vi "Close.vi"(8 "error in (no error)":errorcluster, 11 "NI Digital in":refnum<class "String Out.lvclass">) -> (0 "error out":errorcluster, 3 "NI Digital out":refnum<class "String Out.lvclass">)   [LabVIEW 2018, in "String Out.lvclass"]
doc: "String Out.lvclass:Close.vi\n\nThis is the template for the Close VI for the String Out class.\n\nInstrument Communication Module Version 1.0\nOctober, 2020 Original Code Consulting Daviita Bird\n www.originalcode.com"
uses:
  String Out.lvclass
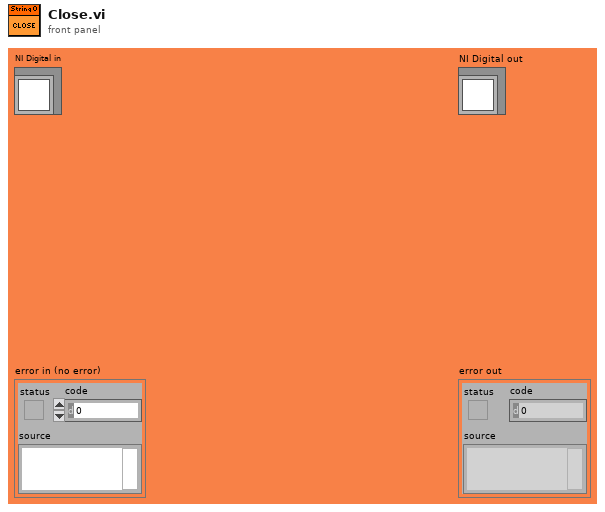
[diagram p1: front panel]
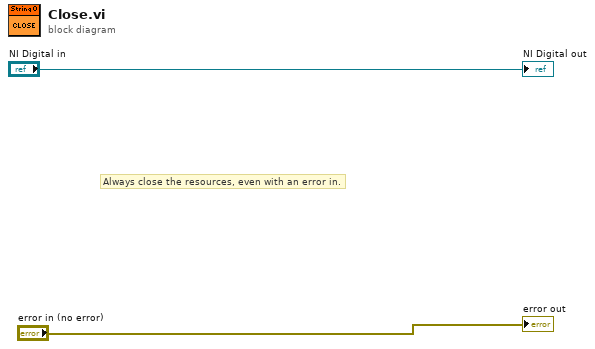
[diagram p0: block diagram]
diagram:
  # "Always close the resources, even with an error in."
  "error out" <- "error in (no error)"
  "NI Digital out" <- "NI Digital in"
